vi "线性公式.vi"(6 "精度":i32=4, 7 "模型":enum32{"线性", "多项式"}(ring), 8 "method":T1 caption="方法" items=["最小二乘", "最小绝对残差", "Bisquare"], 9 "启用":bool[](array[boolean]), 10 "监测浓度":dbl[](array[numeric]), 11 "标液浓度":dbl[](array[numeric])) -> (0 "Polynomial Coefficients":dbl[](array[numeric]) caption="多项式系数", 1 "XY图":cluster{"X Values":dbl[], "Y Values":dbl[]}[](graph), 2 "r^2":dbl format="%.7g", 3 "拟合方程":string)   [LabVIEW 2016, in "总磷总氮曲线模型.xctl"]
uses:
  <vilib>/Analysis/6fits.llb/Curve Fitting Criteria.ctl
  <vilib>/Analysis/NI_AALPro.lvlib
  <vilib>/gmath/NI_Gmath.lvlib
panel:
  out "Best Linear Fit":dbl[](array[numeric]) caption="最佳线性拟合"
  out "二维数组":dbl[][](array[numeric])
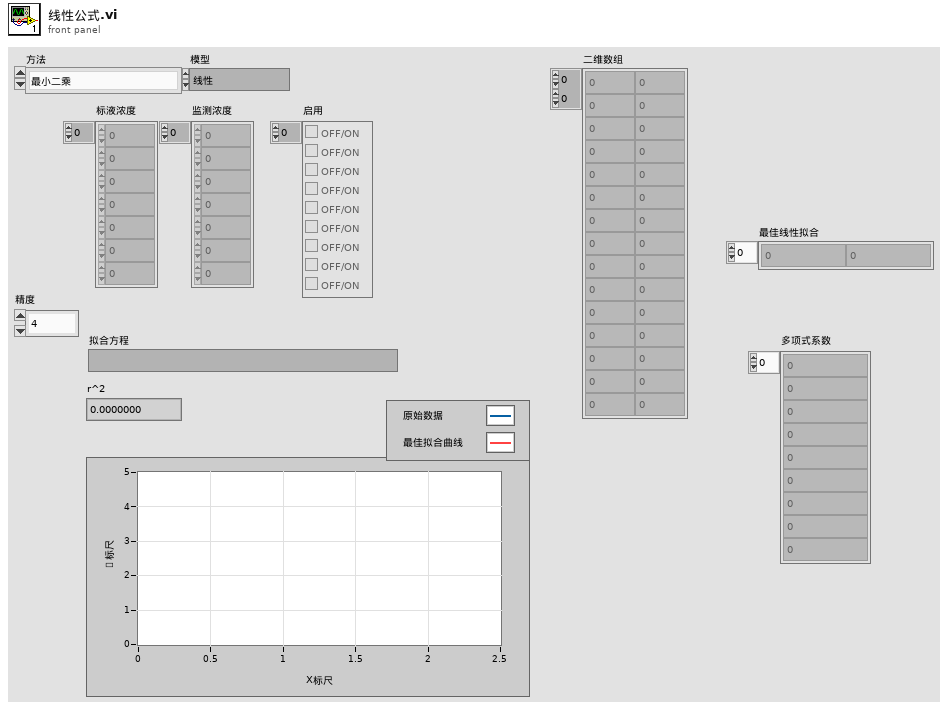
[diagram p1: front panel]
types:
  T1 = typedef "NI_AALPro.lvlib/Curve Fitting Criteria.ctl" = u16
  T2 = enum16{"Linear", "Polynomial", "Exponential", "Power"}
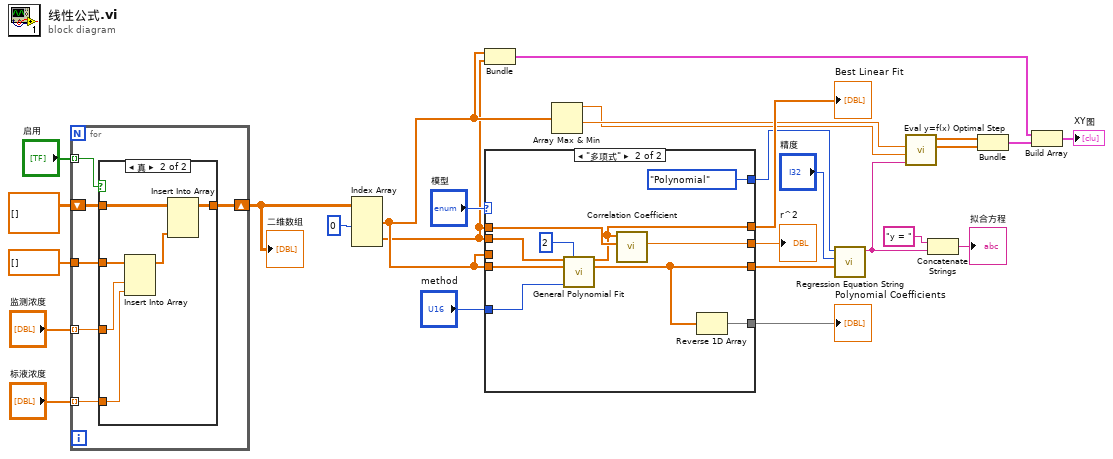
[diagram p0: block diagram]
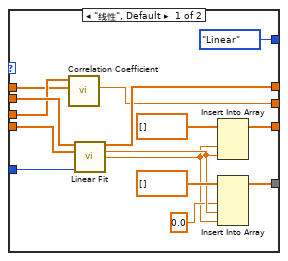
[diagram p2: hidden frame]
diagram:
  n1 = for {
    tunnel: "启用" -> [w28] mode=indexing
    tunnel: "监测浓度" -> [w31] mode=indexing
    tunnel: "标液浓度" -> [w30] mode=indexing
    shift-right: [w29] -> w23
    shift-left: dbl[][] [] ("标液浓度") -> [w33]
    tunnel: dbl[] [] ("监测浓度") -> [w32]
    n2 = case shown="真" w28 {
      tunnel: w33 -> [w34 w40]
      tunnel: w32 -> [_ w39]
      tunnel: w31 -> [_ w38]
      tunnel: w30 -> [_ w37]
      tunnel: [w34 w35] -> w29
      frame False {
      }
      frame True {
        n3 = Insert Into Array(array=w39, new element #1=w38, new element #2=w37) -> (w36:dbl[])  [unwired: 1 in]
        n4 = Insert Into Array(array=w40, new element=w36) -> (w35:dbl[][])  [unwired: 2 in]
      }
    }
  }
  "二维数组" <- w23
  n5 = Index Array(array=w23, index (col) #1=0 ("禁用的索引 (列)")) -> (element #1=w3:dbl[], element #2=w2:dbl[])  [unwired: 3 in]
  n6 = Bundle("标液浓度"=w3, "标液浓度"=w2) -> (w19:cluster{"标液浓度":dbl[], "标液浓度":dbl[]})  [unwired: 1 in]
  n7 = case shown="\"多项式\"" "模型" {
    tunnel: [w55 w59] -> w22
    tunnel: "method" -> [w54 w65]
    tunnel: w3 -> [w51 w61]
    tunnel: w2 -> [w50 w62]
    tunnel: [T2."Linear" ("拟合类型") T2."Polynomial" ("拟合类型")] -> w13
    tunnel: [w53 w57] -> w12
    tunnel: [w49 w58] -> w4
    tunnel: w3 -> [w48 _]
    tunnel: w2 -> [w47 w60]
    tunnel: [w44 w56] -> w1
    frame "线性", Default {
      n8 = call <vilib>:"Correlation Coefficient.vi"("Y"=w47, "X"=w48) -> ("r^2"=w49:dbl)  [unwired: 8 in, 1 out]
      n9 = call <vilib>:"Linear Fit.vi"("Y"=w50, "X"=w51, "method"=w54) -> ("Best Linear Fit"=w55:dbl[], "slope"=w45:dbl, "intercept"=w41:dbl)  [unwired: 8 in, 2 out]
      n10 = Insert Into Array(array=dbl[] [] ("数组"), new element #1=w41, new element #2=w45) -> (w53:dbl[])  [unwired: 1 in]
      n11 = Insert Into Array(array=dbl[] [] ("数组"), new element #1=0.0 ("新元素/子数组"), new element #2=w45, new element #3=w41) -> (w44:dbl[])  [unwired: 1 in]
    }
    frame "多项式" {
      n12 = call <vilib>:"General Polynomial Fit.vi"("Y"=w62, "polynomial order"=2, "X"=w61, "method"=w65) -> ("Best Polynomial Fit"=w59:dbl[], "Polynomial Coefficients"=w57:dbl[])  [unwired: 8 in, 2 out]
      n13 = call <vilib>:"Correlation Coefficient.vi"("Y"=w60, "X"=w59) -> ("r^2"=w58:dbl)  [unwired: 8 in, 1 out]
      n14 = Reverse 1D Array(array=w57) -> (reversed array=w56:dbl[])
    }
  }
  "Best Linear Fit" <- w22
  "r^2" <- w4
  "Polynomial Coefficients" <- w1
  n15 = Array Max & Min(array=w3) -> (max value=w7:dbl, min value=w14:dbl)  [unwired: 2 out]
  n16 = call "Regression Equation String.vi"("系数"=w12, "精度"="精度", "拟合类型"=w13) -> ("公式"=w15:string)  [unwired: 8 in]
  n17 = call <vilib>:"Eval y=f(x) Optimal Step.vi"("formula"=w15, "end"=w7, "start"=w14) -> ("Y Values"=w5:dbl[], "X Values"=w17:dbl[])  [unwired: 2 in, 2 out]
  n18 = Concatenate Strings("y = " ("string"), w15) -> (→"拟合方程":string)
  n19 = Bundle("X Values"=w17, "Y Values"=w5) -> (w18:cluster{"X Values":dbl[], "Y Values":dbl[]})  [unwired: 1 in]
  n20 = Build Array(w19, w18) -> (→"XY图":cluster{"X Values":dbl[], "Y Values":dbl[]}[])
